vi "Vision Processing.vi"(4 "error in (no error)":errorcluster, 7 "Image Size":T1=enum."320x240") -> ()   [LabVIEW 2016]
doc: "This VI runs in parallel to other tasks. It gets images from the camera, processes them for color or shape and use that information to affect robot behavior."
uses:
  <vilib>/Rock Robotics/WPI/Camera/WPI_CameraImageSize.ctl
  <vilib>/Rock Robotics/WPI/Camera/WPI_CameraWhite Balance Values.ctl
  <vilib>/Rock Robotics/WPI/Camera/WPI_CameraExposure Values.ctl
  <vilib>/Rock Robotics/WPI/Camera/WPI_CameraFrameRate.ctl
  Robot Global Data.vi
panel:
  in  "Image Size 2":T1=enum."320x240"
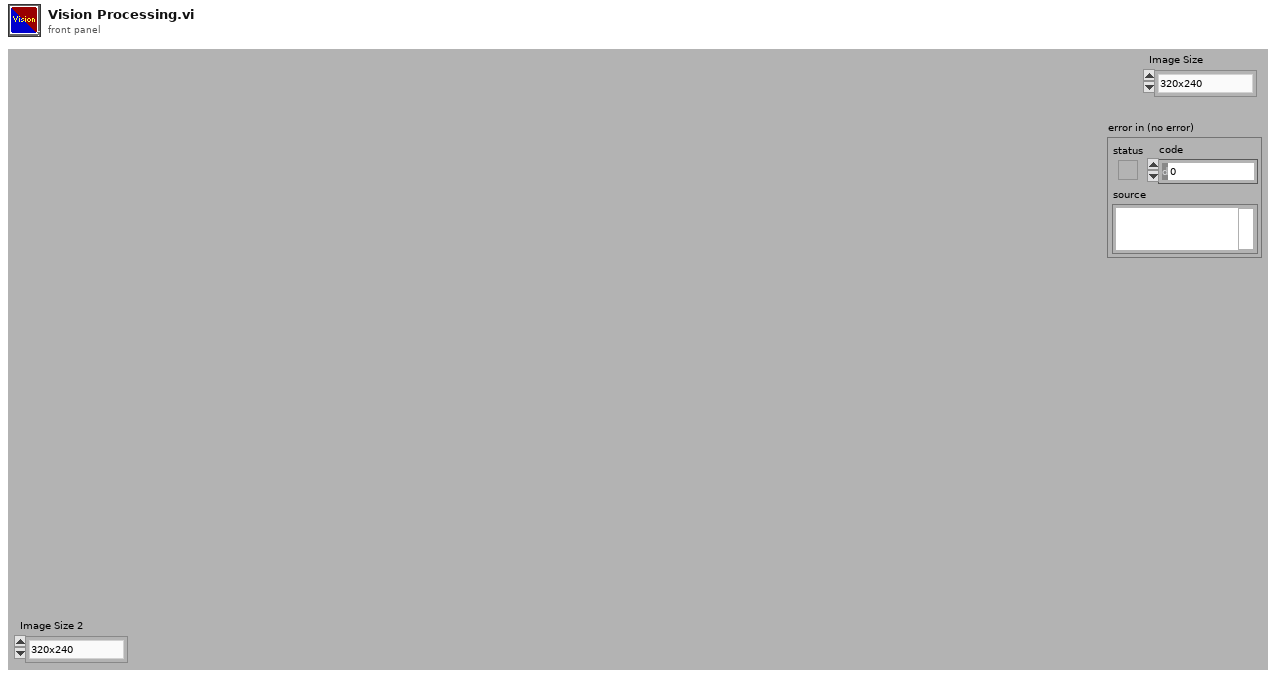
[diagram p1: front panel]
types:
  T1 = typedef "WPI_CameraImageSize.ctl" = enum16{"640x480", "320x240", "160x120", "Custom"}
  T2 = typedef "Image Type" = u32
  T3 = typedef "WPI_CameraFrameRate.ctl" = u32
  T4 = typedef "WPI_CameraExposure Values.ctl" = enum16{"Auto", "Flicker-free 50 Hz", "Flicker-free 60 Hz", "Hold current", "Custom"}
  T5 = typedef "WPI_CameraWhite Balance Values.ctl" = enum16{"Auto", "Fixed indoor", "Fixed outdoor 1", "Fixed outdoor 2", "Fixed fluorescent 1", "Fixed fluorescent 2", "Hold current", "Custom"}
  T6 = typedef "WPI_CameraDevRef.ctl" = cluster{"Camera Address":string, "CameraStatus":errorcluster}
  T7 = typedef "IMAQ Image.ctl" = refnum<image>
  T8 = cluster{"Left":dbl, "Top":dbl, "Right":dbl, "Bottom":dbl}
  T9 = cluster{"Bounding Box Final":cluster{"Left":dbl, "Top":dbl, "Right":dbl, "Bottom":dbl}, "X Resolution":i32, "Y Resolution":i32}
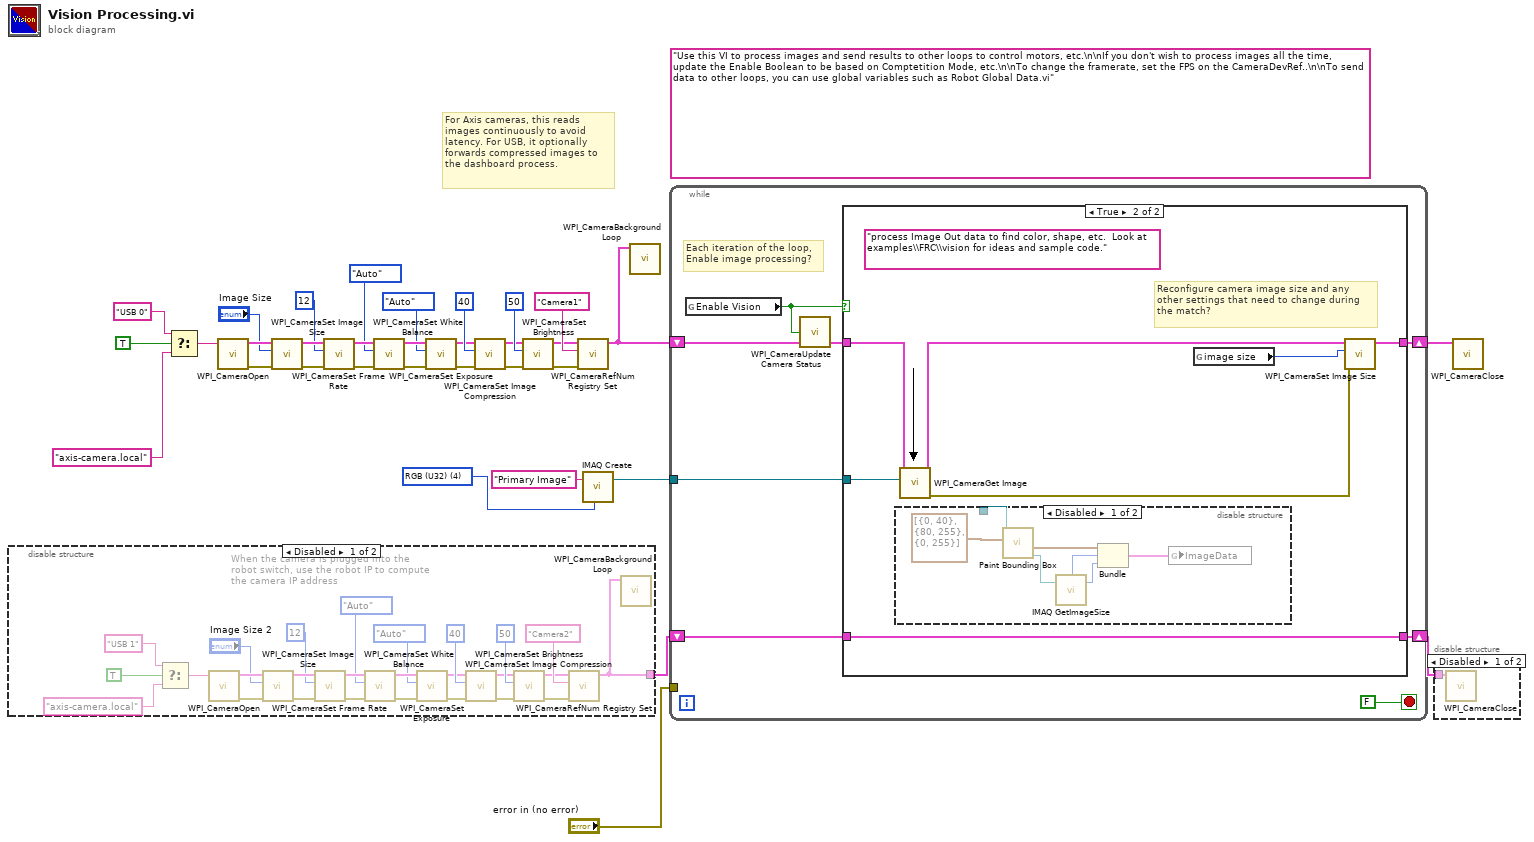
[diagram p0: block diagram]
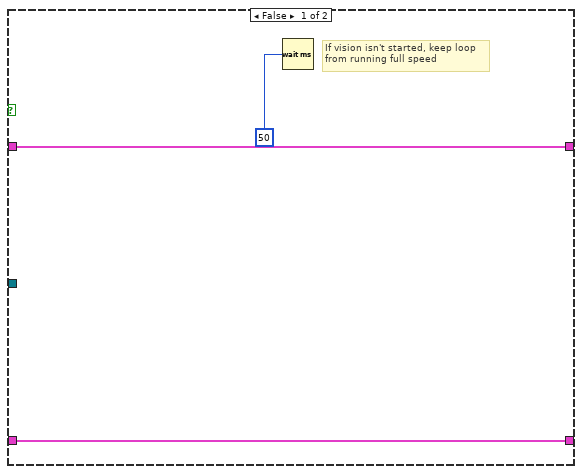
[diagram p4: hidden frame]
diagram:
  w1 = T2 4 items=["Grayscale (U8)", "Grayscale (I16)", "Grayscale (SGL)", "Complex (CSG)", "RGB (U32)", "HSL (U32)", "RGB (U64)"] ("Image Type")
  (unwired) "Use this VI to process images and send results to other loops to control motors, etc.\n\nIf you don't wish to process images all the time, update the Enable Boolean to be based on Comptetition Mode, etc.\n\nTo change the framerate, set the FPS on the CameraDevRef..\n\nTo send data to other loops, you can use global variables such as Robot Global Data.vi"
  # "For Axis cameras, this reads\nimages continuously to avoid\nlatency. For USB, it optionally\nforwards compressed images to\nthe dashboard process."
  n1 = disable-structure shown="Disabled" {
    disable-tunnel: [w59 _] -> w4
    frame Disabled {
      # "When the camera is plugged into the\nrobot switch, use the robot IP to compute\nthe camera IP address"
      n2 = Select(t="USB 1" ("format string"), s=TRUE ("dot notation? (F)"), f="axis-camera.local" ("format string")) -> (s? t:f=w35:string)
      n3 = call <vilib>:"WPI_CameraOpen.vi"("Camera Address"=w35) -> ("error out"=w49:errorcluster, "CameraDevRef"=w50:T6)  [unwired: 1 in, 8 out]
      n4 = call <vilib>:"WPI_CameraSet Image Size.vi"("error in (no error)"=w49, "Image Size"="Image Size 2", "CameraDevRef"=w50) -> ("error out"=w48:errorcluster, "CameraDevRef Out"=w51:T6)  [unwired: 1 in, 6 out]
      n5 = call <vilib>:"WPI_CameraSet Frame Rate.vi"("error in (no error)"=w48, "Frame Rate (fps)"=T3 12, "CameraDevRef"=w51) -> ("error out"=w47:errorcluster, "CameraDevRef Out"=w53:T6)  [unwired: 7 out]
      n6 = call <vilib>:"WPI_CameraSet White Balance.vi"("error in (no error)"=w47, "White Balance"=WPI_CameraWhite_Balance_Values."Auto", "CameraDevRef"=w53) -> ("error out"=w46:errorcluster, "CameraDevRef Out"=w52:T6)  [unwired: 1 in, 6 out]
      n7 = call <vilib>:"WPI_CameraSet Exposure.vi"("error in (no error)"=w46, "Exposure"=WPI_CameraExposure_Values."Auto", "CameraDevRef"=w52) -> ("error out"=w45:errorcluster, "CameraDevRef Out"=w55:T6)  [unwired: 1 in, 6 out]
      n8 = call <vilib>:"WPI_CameraSet Image Compression.vi"("error in (no error)"=w45, "Compression"=40, "CameraDevRef"=w55) -> ("error out"=w44:errorcluster, "CameraDevRef Out"=w54:T6)  [unwired: 7 out]
      n9 = call <vilib>:"WPI_CameraSet Brightness.vi"("error in (no error)"=w44, "Brightness"=50, "CameraDevRef"=w54) -> ("error out"=w42:errorcluster, "CameraDevRef Out"=w43:T6)  [unwired: 7 out]
      n10 = call <vilib>:"WPI_CameraRefNum Registry Set.vi"("error in (no error)"=w42, "refnum name"="Camera2", "CameraDevRef"=w43) -> ("CameraDevRef"=w59:T6)  [unwired: 1 in, 7 out]
      n11 = call <vilib>:"WPI_CameraBackground Loop.vi"("CameraDevRef"=w59) -> ()  [unwired: 11 in]
    }
    frame Enabled {
    }
  }
  n12 = Select(t="USB 0" ("format string"), s=TRUE ("dot notation? (F)"), f="axis-camera.local" ("format string")) -> (s? t:f=w6:string)
  n13 = call <vilib>:"WPI_CameraOpen.vi"("Camera Address"=w6) -> ("error out"=w23:errorcluster, "CameraDevRef"=w24:T6)  [unwired: 1 in, 8 out]
  n14 = call <vilib>:"WPI_CameraSet Image Size.vi"("error in (no error)"=w23, "Image Size"="Image Size", "CameraDevRef"=w24) -> ("error out"=w22:errorcluster, "CameraDevRef Out"=w25:T6)  [unwired: 1 in, 6 out]
  n15 = call <vilib>:"WPI_CameraSet Frame Rate.vi"("error in (no error)"=w22, "Frame Rate (fps)"=T3 12, "CameraDevRef"=w25) -> ("error out"=w21:errorcluster, "CameraDevRef Out"=w27:T6)  [unwired: 7 out]
  n16 = call <vilib>:"WPI_CameraSet White Balance.vi"("error in (no error)"=w21, "White Balance"=WPI_CameraWhite_Balance_Values."Auto", "CameraDevRef"=w27) -> ("error out"=w20:errorcluster, "CameraDevRef Out"=w26:T6)  [unwired: 1 in, 6 out]
  n17 = call <vilib>:"WPI_CameraSet Exposure.vi"("error in (no error)"=w20, "Exposure"=WPI_CameraExposure_Values."Auto", "CameraDevRef"=w26) -> ("error out"=w19:errorcluster, "CameraDevRef Out"=w29:T6)  [unwired: 1 in, 6 out]
  n18 = call <vilib>:"WPI_CameraSet Image Compression.vi"("error in (no error)"=w19, "Compression"=40, "CameraDevRef"=w29) -> ("error out"=w18:errorcluster, "CameraDevRef Out"=w28:T6)  [unwired: 7 out]
  n19 = call <vilib>:"WPI_CameraSet Brightness.vi"("error in (no error)"=w18, "Brightness"=50, "CameraDevRef"=w28) -> ("error out"=w16:errorcluster, "CameraDevRef Out"=w17:T6)  [unwired: 7 out]
  n20 = call <vilib>:"WPI_CameraRefNum Registry Set.vi"("error in (no error)"=w16, "refnum name"="Camera1", "CameraDevRef"=w17) -> ("CameraDevRef"=w12:T6)  [unwired: 1 in, 7 out]
  n21 = call "IMAQ Create"("Image Name"="Primary Image", "Image Type"=w1) -> ("New Image"=w33:T7)  [unwired: 2 in, 2 out]
  n22 = call <vilib>:"WPI_CameraBackground Loop.vi"("CameraDevRef"=w12) -> ()  [unwired: 11 in]
  n23 = while {
    shift-right: [w66] -> w10
    shift-left: w12 -> [w64]
    tunnel: w33 -> [w65]
    tunnel: "error in (no error)" -> [_]
    shift-right: [w60] -> w3
    shift-left: w4 -> [w61]
    stop <- FALSE stop-if-true
    # "Each iteration of the loop,\nEnable image processing?"
    n24 = global read "Robot Global Data.vi" "Enable Vision"() -> (w62:bool)
    n25 = call <vilib>:"WPI_CameraUpdate Camera Status.vi"("CameraDevRef In"=w64, "Enable Vision"=w62) -> ("CameraDevRef Out"=w63:T6)  [unwired: 3 in]
    n26 = case shown="True" w62 {
      tunnel: w65 -> [_ w76]
      tunnel: [w70 w77] -> w66
      tunnel: w63 -> [w70 w74]
      tunnel: w61 -> [w68 w71]
      tunnel: [w68 w71] -> w60
      frame False {
        # "If vision isn't started, keep loop\nfrom running full speed"
        n27 = Wait (ms)(milliseconds to wait=u32 50) -> ()  [unwired: 1 out]
      }
      frame True {
        (unwired) "process Image Out data to find color, shape, etc.  Look at examples\\FRC\\vision for ideas and sample code."
        # "Reconfigure camera image size and any\nother settings that need to change during\nthe match?"
        n28 = disable-structure shown="Disabled" {
          disable-tunnel: _ -> [w84 _]
          frame Disabled {
            n29 = call "Paint Bounding Box.vi"("Camera Image"=w84, "R/G/B"=cluster{"Lower value":i32, "Upper value":i32}[] [{"Lower value"=0, "Upper value"=40}, {"Lower value"=80, "Upper value"=255}, {"Lower value"=0, "Upper value"=255}]) -> ("Thresholded Image"=w81:T7, "Bounding Box Final"=w82:T8)  [unwired: 5 in, 3 out]
            n30 = call "IMAQ GetImageSize"("Image"=w81) -> ("Y Resolution"=w79:i32, "X Resolution"=w80:i32)  [unwired: 3 in, 1 out]
            n31 = Bundle("Bounding Box Final"=w82, "X Resolution"=w80, "Y Resolution"=w79) -> (w78:T9)  [unwired: 1 in]
            n32 = global write "Robot Global Data.vi" "ImageData"(w78) -> ()
          }
          frame Enabled {
          }
        }
        n33 = call <vilib>:"WPI_CameraGet Image.vi"("Image"=w76, "CameraDevRef"=w74) -> ("error out"=w72:errorcluster, "CameraDevRef Out"=w73:T6)  [unwired: 1 in, 7 out]
        n34 = global read "Robot Global Data.vi" "image size"() -> (w75:T1)
        n35 = call <vilib>:"WPI_CameraSet Image Size.vi"("error in (no error)"=w72, "Image Size"=w75, "CameraDevRef"=w73) -> ("CameraDevRef Out"=w77:T6)  [unwired: 1 in, 7 out]
      }
    }
  }
  n36 = disable-structure shown="Disabled" {
    disable-tunnel: w3 -> [w85 _]
    frame Disabled {
      n37 = call <vilib>:"WPI_CameraClose.vi"("CameraDevRef"=w85) -> ()  [unwired: 1 in, 10 out]
    }
    frame Enabled {
    }
  }
  n38 = call <vilib>:"WPI_CameraClose.vi"("CameraDevRef"=w10) -> ()  [unwired: 1 in, 10 out]
